vi "DatabaseFGV.vi"(10 "Set":bool, 11 "State":enum16{"Get", "Set"}(ring)) -> (3 "Active?":bool)   [LabVIEW 2015]
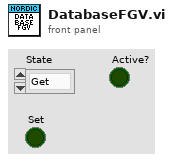
[diagram p1: front panel]
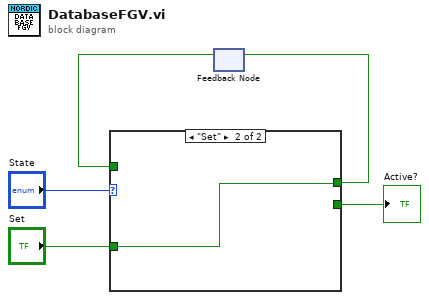
[diagram p0: block diagram]
diagram:
  n1 = feedback #1() -> (w2:bool)  [unwired: 1 in]
  n2 = case shown="\"Set\"" "State" {
    tunnel: "Set" -> [_ w7]
    tunnel: [w6 w7] -> w3
    tunnel: w2 -> [w6 _]
    tunnel: [w6 _] -> w1
    frame "Get", Default {
    }
    frame "Set" {
    }
  }
  "Active?" <- w1
  n3 = feedback-in #1(w3) -> ()
